vi "Separate 4ROI_new2.vi"(0 "ROI Descriptor":T1 {"Contours"."Type" items=["No Selection", "Point", "Line", "Rectangle", "Oval", "Polygon", "Freehand Region", "Annulus", "Unused2", "Unused3", "Broken Line", "Freehand Line", "Rotated Rectangle"]}, 5 "ROIsize":cluster{"Width":dbl, "Height":dbl}[](array[cluster])=[{"Width"=0.375, "Height"=0.2}, {"Width"=0.375, "Height"=0.2}, {"Width"=0.375, "Height"=0.2}, {"Width"=0.375, "Height"=0.2}], 11 "error in":errorcluster) -> (4 "Left ROI":T1 {"Contours"."Type" items=["No Selection", "Point", "Line", "Rectangle", "Oval", "Polygon", "Freehand Region", "Annulus", "Unused2", "Unused3", "Broken Line", "Freehand Line", "Rotated Rectangle"]}, 6 "Top ROI":T1 {"Contours"."Type" items=["No Selection", "Point", "Line", "Rectangle", "Oval", "Polygon", "Freehand Region", "Annulus", "Unused2", "Unused3", "Broken Line", "Freehand Line", "Rotated Rectangle"]}, 8 "Right ROI":T1 {"Contours"."Type" items=["No Selection", "Point", "Line", "Rectangle", "Oval", "Polygon", "Freehand Region", "Annulus", "Unused2", "Unused3", "Broken Line", "Freehand Line", "Rotated Rectangle"]}, 10 "Bottom ROI":T1 {"Contours"."Type" items=["No Selection", "Point", "Line", "Rectangle", "Oval", "Polygon", "Freehand Region", "Annulus", "Unused2", "Unused3", "Broken Line", "Freehand Line", "Rotated Rectangle"]}, 15 "error out":errorcluster)   [LabVIEW 2015]
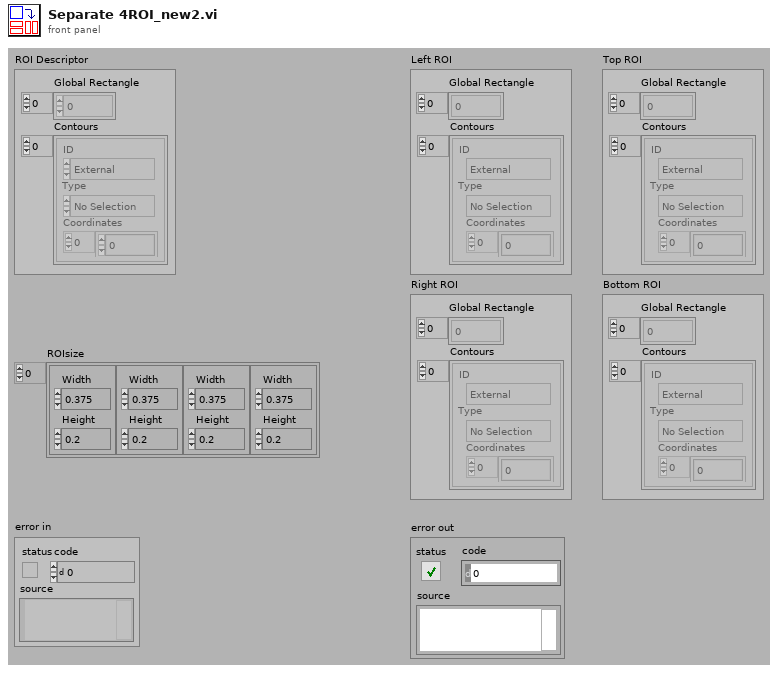
[diagram p1: front panel]
types:
  T1 = typedef "ROI Descriptor" = cluster{"Global Rectangle":i32[], "Contours":cluster{"ID":enum32{"External", "Internal"}, "Type":u32, "Coordinates":i32[]}[]}
  T2 = typedef "IMAQ Rectangle" = cluster{"Left":i32, "Top":i32, "Right":i32, "Bottom":i32, "Rotation":dbl}
  T3 = typedef "IMAQ Point" = cluster{"X":sgl, "Y":sgl}
  T4 = cluster{"HorizontalWidth":dbl, "HorizontalHeight":dbl}
  T5 = cluster{"VerticalWidth":dbl, "VerticalHeight":dbl}
  T6 = cluster{"MiddleRight_X":dbl, "MiddleRight_Y":dbl}
  T7 = cluster{"MiddleBottom_X":dbl, "MiddleBottom_Y":dbl}
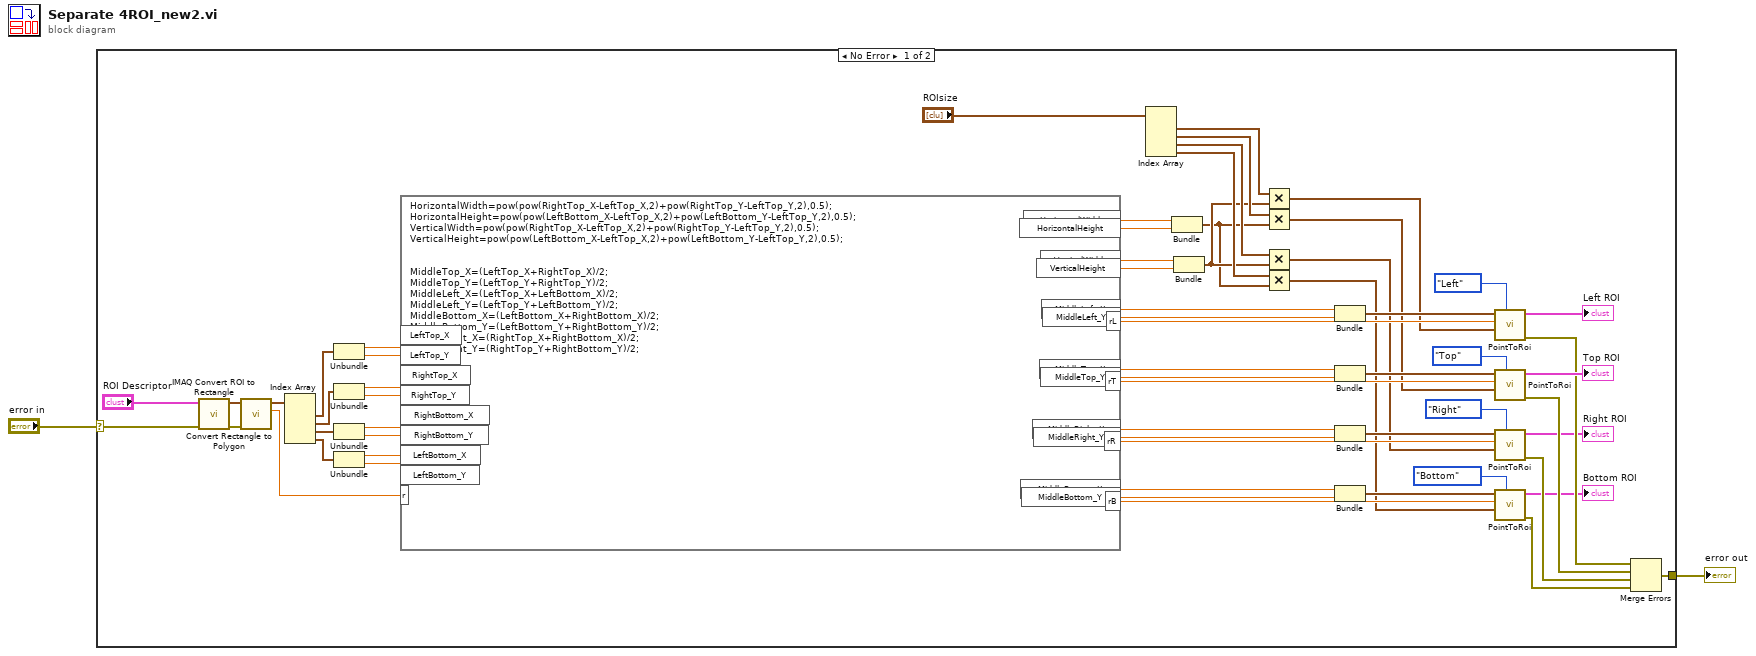
[diagram p0: block diagram]
diagram:
  n1 = case shown="No Error" "error in" {
    selector: "error in" -> [w24 w65]
    tunnel: [w25 w65] -> w2
    frame No Error {
      n2 = call "IMAQ Convert ROI to Rectangle"("error in (no error)"=w24, "ROI Descriptor"="ROI Descriptor") -> ("error out"=w33:errorcluster, "Rectangle"=w36:T2)  [unwired: 7 in]
      n3 = call "Convert Rectangle to Polygon.vi"("error in (no error)"=w33, "Rectangle"=w36) -> ("Rotation"=w34:dbl, "Rectangle Points"=w35:T3[])  [unwired: 7 in, 1 out]
      n4 = Index Array(array=w35) -> (element #1=w43:T3, element #2=w42:T3, element #3=w64:T3, element #4=w44:T3)  [unwired: 4 in]
      n5 = Unbundle(w43) -> ("X"=w63:sgl, "Y"=w62:sgl)
      n6 = Unbundle(w42) -> ("X"=w61:sgl, "Y"=w60:sgl)
      n7 = Unbundle(w64) -> ("X"=w59:sgl, "Y"=w58:sgl)
      n8 = Unbundle(w44) -> ("X"=w57:sgl, "Y"=w56:sgl)
      n9 = formula code="HorizontalWidth=pow(pow(RightTop_X-LeftTop_X,2)+pow(RightTop_Y-LeftTop_Y,2),0.5);\nHorizontalHeight=pow(pow(LeftBottom_X-LeftTop_X,2)+pow(LeftBottom_Y-LeftTop_Y,2),0.5);\nVerticalWidth=pow(pow(RightTop_X-LeftTop_X,2)+pow(RightTop_Y-LeftTop_Y,2),0.5);\nVerticalHeight=pow(pow(LeftBottom_X-LeftTop_X,2)+pow(LeftBottom_Y-LeftTop_Y,2),0.5);\n\n\nMiddleTop_X=(LeftTop_X+RightTop_X)/2;\nMiddleTop_Y=(LeftTop_Y+RightTop_Y)/2;\nMiddleLeft_X=(LeftTop_X+LeftBottom_X)/2;\nMiddleLeft_Y=(LeftTop_Y+LeftBottom_Y)/2;\nMiddleBottom_X=(LeftBottom_X+RightBottom_X)/2;\nMiddleBottom_Y=(LeftBottom_Y+RightBottom_Y)/2;\nMiddleRight_X=(RightTop_X+RightBottom_X)/2;\nMiddleRight_Y=(RightTop_Y+RightBottom_Y)/2;\n\n\nrL=r+90;\nrT=r+0;\nrR=r+270;\nrB=r+180;"("LeftTop_X"=w63, "LeftTop_Y"=w62, "RightTop_X"=w61, "RightTop_Y"=w60, "RightBottom_X"=w59, "RightBottom_Y"=w58, "LeftBottom_X"=w57, "LeftBottom_Y"=w56, "r"=w34) -> ("MiddleTop_X"=w55:dbl, "MiddleTop_Y"=w54:dbl, "MiddleLeft_X"=w53:dbl, "MiddleLeft_Y"=w52:dbl, "MiddleRight_X"=w51:dbl, "MiddleRight_Y"=w50:dbl, "MiddleBottom_X"=w49:dbl, "MiddleBottom_Y"=w48:dbl, "rT"=w37:dbl, "rL"=w38:dbl, "rR"=w39:dbl, "rB"=w40:dbl, "HorizontalWidth"=w16:dbl, "HorizontalHeight"=w17:dbl, "VerticalWidth"=w4:dbl, "VerticalHeight"=w3:dbl)
      n10 = Index Array(array="ROIsize") -> (element #1=w10:cluster{"Width":dbl, "Height":dbl}, element #2=w9:cluster{"Width":dbl, "Height":dbl}, element #3=w8:cluster{"Width":dbl, "Height":dbl}, element #4=w7:cluster{"Width":dbl, "Height":dbl})  [unwired: 4 in]
      n11 = Bundle("HorizontalWidth"=w16, "HorizontalHeight"=w17) -> (w5:T4)  [unwired: 1 in]
      n12 = Bundle("VerticalWidth"=w4, "VerticalHeight"=w3) -> (w6:T5)  [unwired: 1 in]
      n13 = Multiply(x=w10, y=w6) -> (x*y=w14:cluster{dbl, dbl})
      n14 = Multiply(x=w9, y=w5) -> (x*y=w13:cluster{dbl, dbl})
      n15 = Multiply(x=w8, y=w6) -> (x*y=w12:cluster{dbl, dbl})
      n16 = Multiply(x=w7, y=w5) -> (x*y=w11:cluster{dbl, dbl})
      n17 = Bundle("MiddleLeft_X"=w53, "MiddleLeft_Y"=w52) -> (w47:cluster{"MiddleLeft_X":dbl, "MiddleLeft_Y":dbl})  [unwired: 1 in]
      n18 = Bundle("MiddleTop_X"=w55, "MiddleTop_Y"=w54) -> (w32:cluster{"MiddleTop_X":dbl, "MiddleTop_Y":dbl})  [unwired: 1 in]
      n19 = Bundle("MiddleRight_X"=w51, "MiddleRight_Y"=w50) -> (w46:T6)  [unwired: 1 in]
      n20 = Bundle("MiddleBottom_X"=w49, "MiddleBottom_Y"=w48) -> (w45:T7)  [unwired: 1 in]
      n21 = call "PointToRoi.vi"("Director"=enum16{"Left", "Top", "Right", "Bottom"}."Left", "ROISize"=w14, "r"=w38, "Point"=w47) -> ("error out"=w29:errorcluster, "ROI Descriptor"=→"Left ROI":T1)  [unwired: 6 in]
      n22 = call "PointToRoi.vi"("Director"=enum16{"Left", "Top", "Right", "Bottom"}."Top", "ROISize"=w13, "r"=w37, "Point"=w32) -> ("error out"=w28:errorcluster, "ROI Descriptor"=→"Top ROI":T1)  [unwired: 6 in]
      n23 = call "PointToRoi.vi"("Director"=enum16{"Left", "Top", "Right", "Bottom"}."Right", "ROISize"=w12, "r"=w39, "Point"=w46) -> ("error out"=w27:errorcluster, "ROI Descriptor"=→"Right ROI":T1)  [unwired: 6 in]
      n24 = call "PointToRoi.vi"("Director"=enum16{"Left", "Top", "Right", "Bottom"}."Bottom", "ROISize"=w11, "r"=w40, "Point"=w45) -> ("error out"=w26:errorcluster, "ROI Descriptor"=→"Bottom ROI":T1)  [unwired: 6 in]
      n25 = Merge Errors(w29, w28, w27, w26) -> (w25:errorcluster)
    }
    frame Error {
    }
  }
  "error out" <- w2
